vi "DAQmx Read (Counter DBL 1Chan 1Samp).vi"(0 "task/channels in":refnum<k21>, 9 "timeout":dbl=10.0 format="%0.2f", 11 "error in":errorcluster) -> (4 "task out":refnum<k21>, 6 "data":dbl format="%0.2f", 15 "error out":errorcluster)   [LabVIEW 2013]
doc: "Reads a single floating-point sample from a counter task. Use an instance that reads floating-point values when NI-DAQmx scales counter samples to a floating-point value, such as for frequency and period measurement."
uses:
  nilvaiu.dll
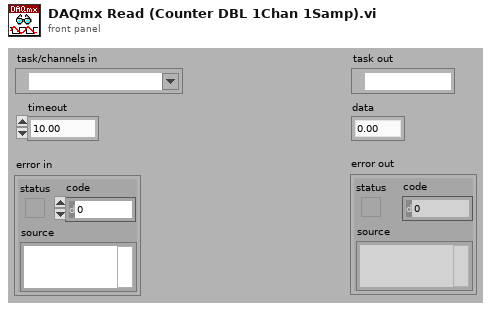
[diagram p1: front panel]
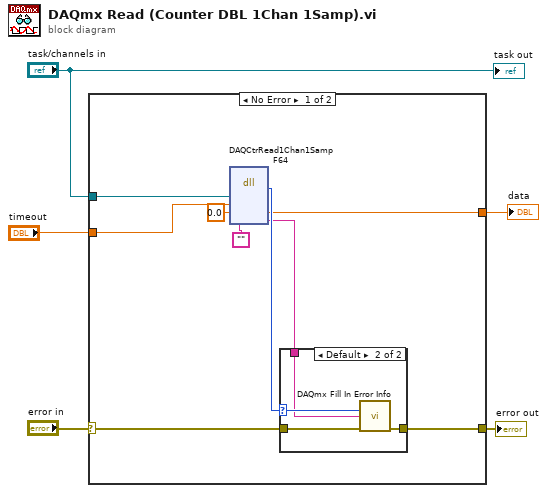
[diagram p0: block diagram]
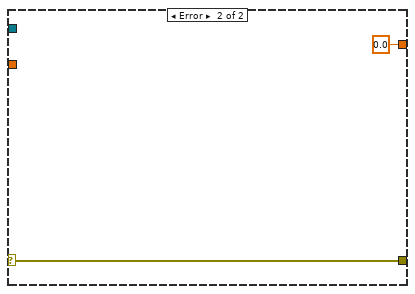
[diagram p3: hidden frame]
diagram:
  n1 = case shown="No Error" "error in" {
    selector: "error in" -> [w7 w20]
    tunnel: [w12 w20] -> w4
    tunnel: "task/channels in" -> [w14 _]
    tunnel: [w8 0.0 ("data")] -> w2
    tunnel: "timeout" -> [w6 _]
    frame No Error {
      n2 = dll-call lib="nilvaiu.*" fn="DAQCtrRead1Chan1SampF64"("taskID"=w14, "timeout"=w6, "data"=0.0, "extendedErrorInfo"="") -> (w13:i32, "data"=w8:dbl, "extendedErrorInfo"=w10:string)  [unwired: 4 in, 3 out]
      n3 = case shown="Default" w13 {
        selector: w13 -> [_ w17]
        tunnel: w7 -> [w15 w19]
        tunnel: [w15 w18] -> w12
        tunnel: w10 -> [_ w16]
        frame 0 {
        }
        frame Default {
          n4 = call "DAQmx Fill In Error Info.vi"("status code"=w17, "extended error info"=w16, "error in"=w19) -> ("error out"=w18:errorcluster)  [unwired: 1 in, 11 out]
        }
      }
    }
    frame Error {
    }
  }
  "error out" <- w4
  "data" <- w2
  "task out" <- "task/channels in"
